vi "tree_control_plot.vi"(8 "Point":T1, 9 "Plot Tree":refnum<vi>, 10 "Output File Loaded?":refnum<vi>) -> ()   [LabVIEW 2019]
uses:
  <vilib>/Utility/miscctls.llb/LVPositionTypeDef.ctl
panel:
  out "Blue":u32
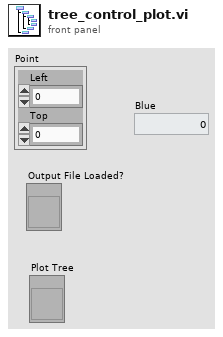
[diagram p1: front panel]
types:
  T1 = typedef "LVPositionTypeDef.ctl" = cluster{"Left":i32, "Top":i32}
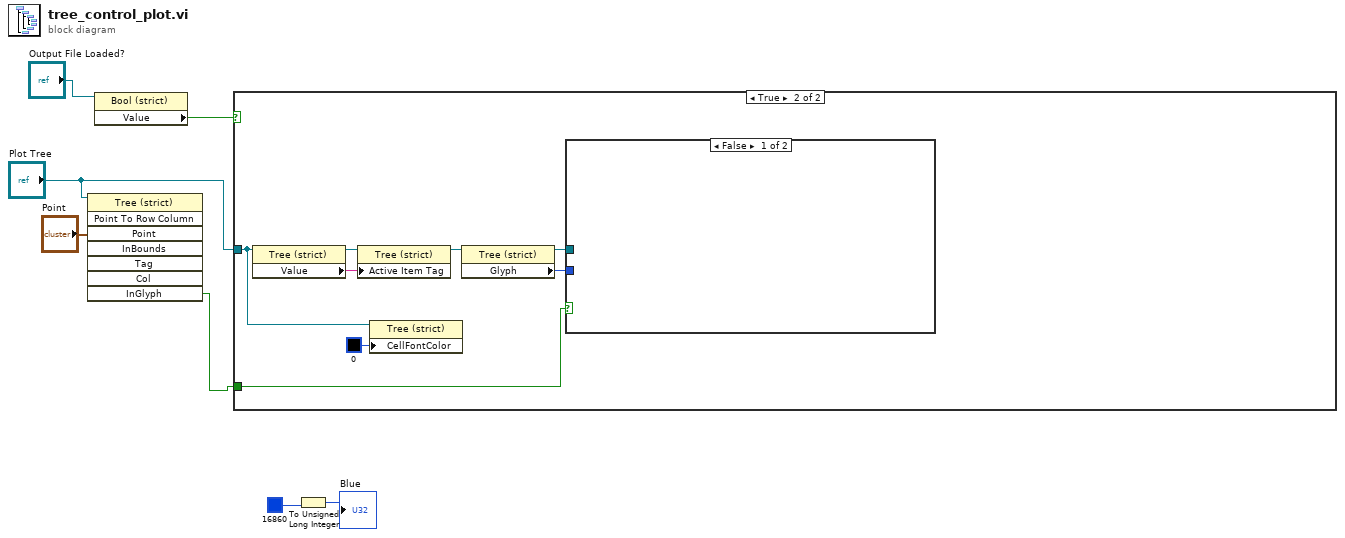
[diagram p0: block diagram]
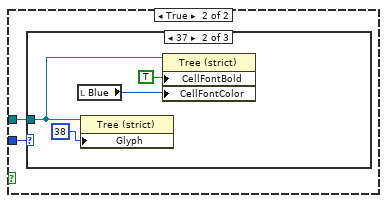
[diagram p3: hidden frame]
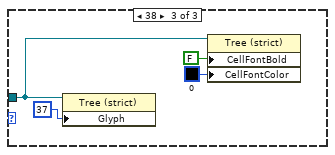
[diagram p5: hidden frame]
diagram:
  n1 = invoke on="Invoke Node" class="Tree (strict)" method="Point To Row Column"(reference="Plot Tree", "Point"="Point") -> ("InGlyph"=w6:bool)  [unwired: 6 in, 7 out]
  n2 = property class="Bool (strict)"(reference="Output File Loaded?") -> ("Value"=w3:bool)  [unwired: 1 in, 2 out]
  n3 = case shown="True" w3 {
    tunnel: "Plot Tree" -> [_ w15]
    tunnel: w6 -> [_ w14]
    frame False {
    }
    frame True {
      n4 = property on="Property Node" class="Tree (strict)"(reference=w15) -> (reference out=w12:refnum<vi>, "Value"=w13:string)  [unwired: 1 in, 1 out]
      n5 = property on="Property Node" class="Tree (strict)"(reference=w12, "Active Item Tag"=w13) -> (reference out=w11:refnum<vi>)  [unwired: 1 in, 1 out]
      n6 = property class="Tree (strict)"(reference=w15, "CellFontColor"=u32 0 ("Active Cell:Cell Font:Color")) -> ()  [unwired: 1 in, 2 out]
      n7 = property on="Property Node" class="Tree (strict)"(reference=w11) -> (reference out=w10:refnum<vi>, "Glyph"=w9:i32)  [unwired: 1 in, 1 out]
      n8 = case shown="False" w14 {
        tunnel: w10 -> [_ w17]
        tunnel: w9 -> [_ w16]
        frame False {
        }
        frame True {
          n9 = case shown="37" w16 {
            tunnel: w17 -> [_ w20 w24]
            frame 15, Default {
            }
            frame 37 {
              n10 = local read "Blue"() -> (w18:u32)
              n11 = property on="Property Node" class="Tree (strict)"(reference=w20, "Glyph"=38 ("Active Item:Symbol Index")) -> ()  [unwired: 1 in, 2 out]
              n12 = property class="Tree (strict)"(reference=w20, "CellFontBold"=TRUE ("Active Cell:Cell Font:Bold"), "CellFontColor"=w18) -> ()  [unwired: 1 in, 2 out]
            }
            frame 38 {
              n13 = property on="Property Node" class="Tree (strict)"(reference=w24, "Glyph"=37 ("Active Item:Symbol Index")) -> ()  [unwired: 1 in, 2 out]
              n14 = property class="Tree (strict)"(reference=w24, "CellFontBold"=FALSE ("Active Cell:Cell Font:Bold"), "CellFontColor"=u32 0 ("Active Cell:Cell Font:Color")) -> ()  [unwired: 1 in, 2 out]
            }
          }
        }
      }
    }
  }
  n15 = To Unsigned Long Integer(number=u32 16860) -> (unsigned 32bit integer=→"Blue":u32)
